vi "frequency-field relation.vi"() -> ()   [LabVIEW 2017]
panel:
  out "f_res":dbl[unit]
  out "B_res":dbl[unit]
  out "SiC Bres_high":dbl[unit]
  out "SiC Bres_low":dbl[unit]
  in  "SiC freq":dbl[unit]
  out "SiC fres_high":dbl[unit]
  out "SiC fres_low":dbl[unit]
  in  "SiC field":dbl[unit]
  in  "SiC zero field state splitting = 2D\n(peak splitting = 4D)":dbl[unit]=68000000.0
  in  "SiC g-factor":dbl=2.008
  in  "h":dbl[unit]=6.62607015e-34
  in  "mu_B":dbl[unit]=9.274009994e-24
  in  "stop":bool
  in  "g-factor":dbl=2.0
  in  "Magnetic Field":dbl[unit]=0.31315185321917494
  in  "Frequency":dbl[unit]=8765900000.0
  # "S=3/2 Zeeman effect (e.g. SiC)"
  # "Simple S=1/2 Zeeman effect"
  # "Changing the left values will change the right values"
  # "Changing the left values will change the right values"
  # "Parameter for spin 1/2 system"
  # "Constants"
  # "Parameters for spin 3/2 system"
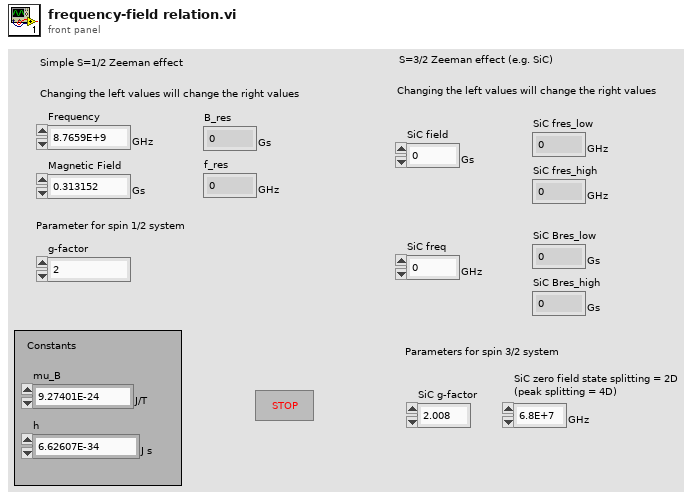
[diagram p1: front panel]
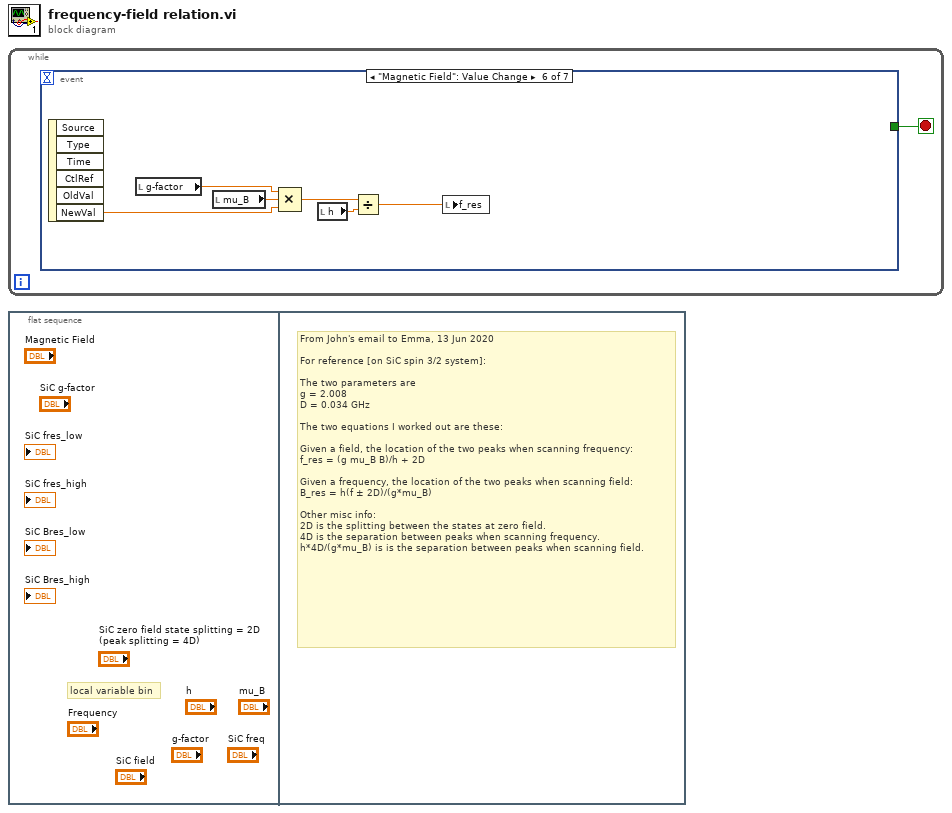
[diagram p0: block diagram]
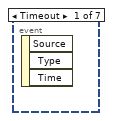
[diagram p2: hidden frame]
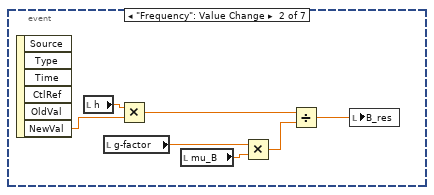
[diagram p3: hidden frame]
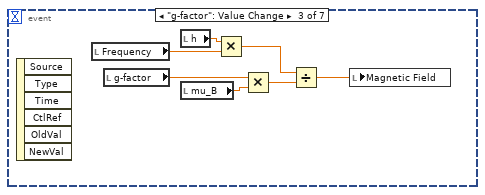
[diagram p4: hidden frame]
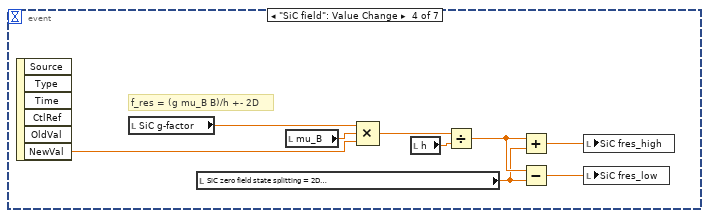
[diagram p5: hidden frame]
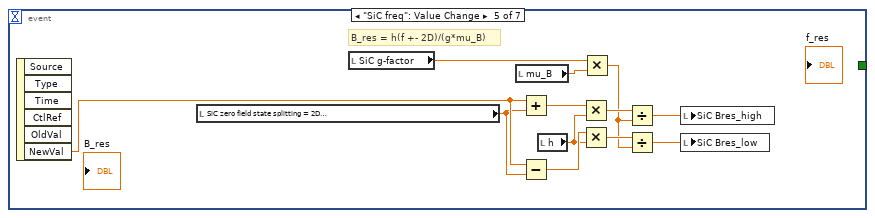
[diagram p6: hidden frame]
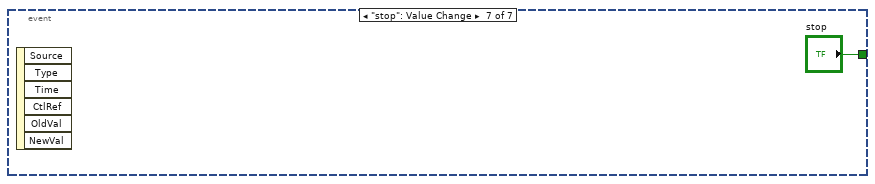
[diagram p7: hidden frame]
diagram:
  n1 = while {
    stop <- w1 stop-if-true
    n2 = event shown="[5] \"Magnetic Field\": Value Change" {
      selector: _ -> [_ _ _ _ _ _ _]
      dyn-events: _ -> [_ _ _ _ _ _ _]
      timeout: _ -> [_ _ _ _ _ _ _]
      tunnel: [_ _ _ _ _ _ "stop"] -> w1
      event Timeout {
        n3 = event-data() -> ()  [unwired: 1 in, 3 out]
      }
      event "Frequency": Value Change {
        n4 = event-data() -> ("NewVal"=w2:dbl[unit])  [unwired: 1 in, 5 out]
        n5 = local read "h"() -> (w8:dbl[unit])
        n6 = local read "g-factor"() -> (w7:dbl)
        n7 = Multiply(x=w8, y=w2) -> (x*y=w4:dbl[unit])
        n8 = local read "mu_B"() -> (w6:dbl[unit])
        n9 = Multiply(x=w7, y=w6) -> (x*y=w5:dbl[unit])
        n10 = Divide(x=w4, y=w5) -> (x/y=w3:dbl[unit])
        n11 = local write "B_res"(w3) -> ()
      }
      event "g-factor": Value Change {
        n12 = event-data() -> ()  [unwired: 1 in, 6 out]
        n13 = local read "Frequency"() -> (w14:dbl[unit])
        n14 = local read "g-factor"() -> (w13:dbl)
        n15 = local read "h"() -> (w15:dbl[unit])
        n16 = local read "mu_B"() -> (w12:dbl[unit])
        n17 = Multiply(x=w15, y=w14) -> (x*y=w10:dbl[unit])
        n18 = Multiply(x=w13, y=w12) -> (x*y=w11:dbl[unit])
        n19 = Divide(x=w10, y=w11) -> (x/y=w9:dbl[unit])
        n20 = local write "Magnetic Field"(w9) -> ()
      }
      event "SiC field": Value Change {
        # "f_res = (g mu_B B)/h +- 2D"
        n21 = event-data() -> ("NewVal"=w20:dbl[unit])  [unwired: 1 in, 5 out]
        n22 = local read "SiC g-factor"() -> (w22:dbl)
        n23 = local read "SiC zero field state splitting = 2D\n(peak splitting = 4D)"() -> (w18:dbl[unit])
        n24 = local read "mu_B"() -> (w21:dbl[unit])
        n25 = Compound Arithmetic op=MULTIPLY(w22, w21, w20) -> (w24:dbl[unit])
        n26 = local read "h"() -> (w23:dbl[unit])
        n27 = Divide(x=w24, y=w23) -> (x/y=w19:dbl[unit])
        n28 = Add(x=w19, y=w18) -> (x+y=w17:dbl[unit])
        n29 = Subtract(x=w19, y=w18) -> (x-y=w16:dbl[unit])
        n30 = local write "SiC fres_high"(w17) -> ()
        n31 = local write "SiC fres_low"(w16) -> ()
      }
      event "SiC freq": Value Change {
        # "B_res = h(f +- 2D)/(g*mu_B)"
        n32 = event-data() -> ("NewVal"=w36:dbl[unit])  [unwired: 1 in, 5 out]
        n33 = local read "SiC zero field state splitting = 2D\n(peak splitting = 4D)"() -> (w35:dbl[unit])
        n34 = local read "SiC g-factor"() -> (w29:dbl)
        n35 = local read "mu_B"() -> (w28:dbl[unit])
        n36 = Add(x=w36, y=w35) -> (x+y=w33:dbl[unit])
        n37 = Subtract(x=w36, y=w35) -> (x-y=w34:dbl[unit])
        n38 = local read "h"() -> (w32:dbl[unit])
        n39 = Multiply(x=w33, y=w32) -> (x*y=w30:dbl[unit])
        n40 = Multiply(x=w34, y=w32) -> (x*y=w31:dbl[unit])
        n41 = Multiply(x=w29, y=w28) -> (x*y=w27:dbl[unit])
        n42 = Divide(x=w30, y=w27) -> (x/y=w26:dbl[unit])
        n43 = Divide(x=w31, y=w27) -> (x/y=w25:dbl[unit])
        n44 = local write "SiC Bres_high"(w26) -> ()
        n45 = local write "SiC Bres_low"(w25) -> ()
      }
      event "Magnetic Field": Value Change {
        n46 = event-data() -> ("NewVal"=w37:dbl[unit])  [unwired: 1 in, 5 out]
        n47 = local read "g-factor"() -> (w41:dbl)
        n48 = local read "mu_B"() -> (w42:dbl[unit])
        n49 = Compound Arithmetic op=MULTIPLY(w41, w42, w37) -> (w40:dbl[unit])
        n50 = local read "h"() -> (w39:dbl[unit])
        n51 = Divide(x=w40, y=w39) -> (x/y=w38:dbl[unit])
        n52 = local write "f_res"(w38) -> ()
      }
      event "stop": Value Change {
        n53 = event-data() -> ()  [unwired: 1 in, 6 out]
      }
    }
  }
  n54 = flat-sequence {
    frame #0 {
      # "local variable bin"
    }
    frame #1 {
      # "From John's email to Emma, 13 Jun 2020\n\nFor reference [on SiC spin 3/2 system]:\n\nThe two parameters are\ng = 2.008\nD = 0.034 GHz\n\nThe two equations I worked out are these:\n\nGiven a field, the location of the two peaks when scanning frequency:\nf_res = (g mu_B B)/h + 2D\n\nGiven a frequency, the location of the two peaks when scanning field: \nB_res = h(f ± 2D)/(g*mu_B)\n\nOther misc info:\n2D is the splitting between the states at zero field.\n4D is the separation between peaks when scanning frequency.\nh*4D/(g*mu_B) is is the separation between peaks when scanning field."
    }
  }
